vi "OAT Kaiser Parameters.vi"(8 "A stop [dB]":dbl=72.0 format="%.2f", 10 "delta f":dbl=0.1 format="%.2f", 11 "fs":dbl=1.0 format="%.2f") -> (0 "beta":dbl format="%.2f", 3 "taps":i32)   [LabVIEW 2017, in "SoundVib_Resampling.lvlib"]
uses:
  <vilib>/addons/Sound and Vibration/Order Analysis/Resample Order Tracking/SoundVib_Resampling.lvlib
  <vilib>/addons/Sound and Vibration/Order Analysis/Referece Data Processing/SoundVib_RefDataProcess.lvlib
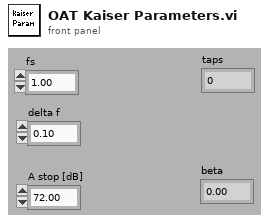
[diagram p1: front panel]
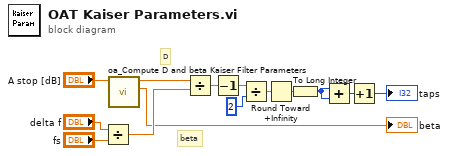
[diagram p0: block diagram]
diagram:
  # "D"
  # "beta"
  n1 = Divide(x="delta f", y="fs") -> (x/y=w9:dbl)
  n2 = call <vilib>:"oa_Compute D and beta Kaiser Filter Parameters.vi"("A stop"="A stop [dB]") -> ("beta"=→"beta":dbl, "D"=w2:dbl)  [unwired: 9 in]
  n3 = Divide(x=w2, y=w9) -> (x/y=w8:dbl)
  n4 = Decrement(x=w8) -> (x-1=w4:dbl)
  n5 = Divide(x=w4, y=2) -> (x/y=w12:dbl)
  n6 = Round Toward +Infinity(x=w12) -> (ceil(x): smallest int >= x=w13:dbl)
  n7 = To Long Integer(number=w13) -> (32bit integer=w6:i32)
  n8 = Add(x=w6, y=w6) -> (x+y=w7:i32)
  n9 = Increment(x=w7) -> (x+1=→"taps":i32)
